vi "return error info.vi"(11 "Error in":refnum<class>) -> (0 "Report Error":bool, 1 "Severity":T1, 2 "Error Location":refnum<class>, 3 "Error to Process":errorcluster)   [LabVIEW 2020, in "Error Interface.lvlib" / "Error.lvclass"]
uses:
  Error.lvclass
  typedefs/error severity.ctl
  Error.lvclass/Error.ctl
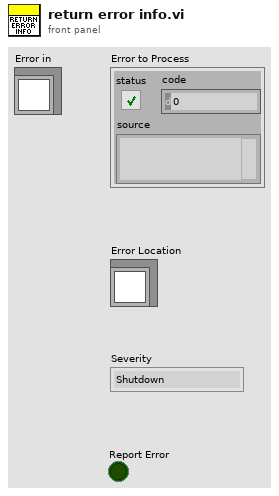
[diagram p1: front panel]
types:
  T1 = typedef "Error Interface.lvlib/Error.lvclass/error severity.ctl" = enum16{"Shutdown", "Restart Calling Actor", "Restart Nested Actor", "Do Nothing"}
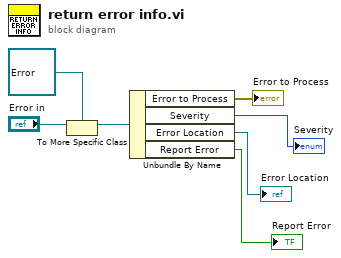
[diagram p0: block diagram]
diagram:
  n1 = To More Specific Class(target class=refnum<class "Error.lvclass"> refnum ("Error in"), reference="Error in") -> (specific class reference=w3:refnum<class "Error.lvclass">)  [unwired: 1 in, 1 out]
  n2 = Unbundle By Name(w3) -> ("Error to Process"=→"Error to Process":errorcluster, "Severity"=→"Severity":T1, "Error Location"=→"Error Location":refnum<class>, "Report Error"=→"Report Error":bool)
